vi "Read VeriSTAND Channel Info.vi"(8 "error in (no error)":errorcluster, 11 "ChannelVS in":refnum<class "ChannelVS.lvclass">) -> (0 "error out":errorcluster, 1 "VeriSTAND Reference":T1=18446744073709551615 format="%.0x", 2 "Exist in VeriSTAND":bool, 3 "ChannelVS out":refnum<class "ChannelVS.lvclass">, 4 "Supported in CD":bool)   [LabVIEW 2020, in "Shared Variables CD 2.0 Configuration.lvlib" / "ChannelVS.lvclass"]
uses:
  ChannelVS.lvclass
  <vilib>/NI VeriStand/Custom Device API/Custom Device Item Ref.ctl
  ChannelVS.lvclass/ChannelVS.ctl
  <vilib>/NI VeriStand/Custom Device API/Custom Device API.lvlib
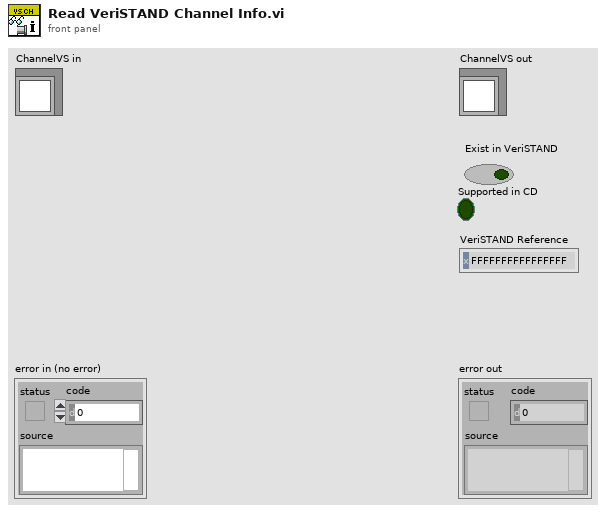
[diagram p1: front panel]
types:
  T1 = typedef "Custom Device API.lvlib/Custom Device Item Ref.ctl" = u64
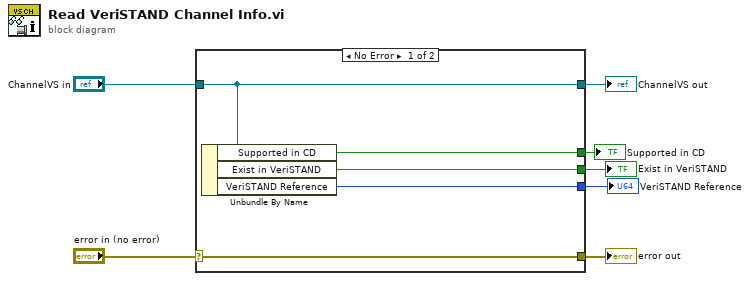
[diagram p0: block diagram]
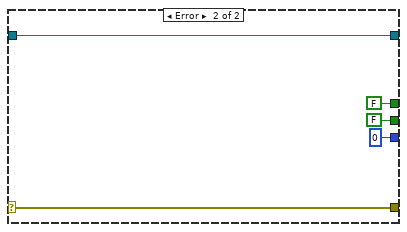
[diagram p2: hidden frame]
diagram:
  n1 = case shown="No Error" "error in (no error)" {
    selector: "error in (no error)" -> [w12 w16]
    tunnel: [w12 w16] -> w6
    tunnel: [w11 w17] -> w4
    tunnel: "ChannelVS in" -> [w11 w17]
    tunnel: [w10 FALSE ("Exist in VeriSTAND")] -> w3
    tunnel: [w9 T1 0 ("VeriSTAND Reference")] -> w2
    tunnel: [w8 FALSE ("Supported in CD")] -> w1
    frame No Error {
      n2 = Unbundle By Name(w11) -> ("Supported in CD"=w8:bool, "Exist in VeriSTAND"=w10:bool, "VeriSTAND Reference"=w9:T1)
    }
    frame Error {
    }
  }
  "error out" <- w6
  "ChannelVS out" <- w4
  "Exist in VeriSTAND" <- w3
  "VeriSTAND Reference" <- w2
  "Supported in CD" <- w1
